vi "Binary Multiplication.vi"(10 "NUM 2 (Binary)":i32 format="%b", 11 "NUM 1 (Binary)":i32 format="%b") -> (3 "PRODUCT  (Binary)":i32 format="%b")   [LabVIEW 2020]
doc: "This VI will find a product between two Binary Numbers."
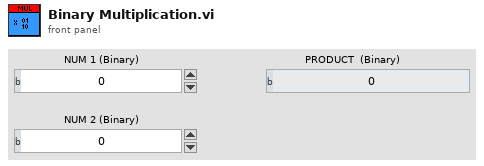
[diagram p1: front panel]
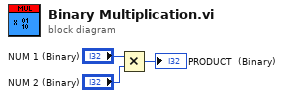
[diagram p0: block diagram]
diagram:
  n1 = Multiply(x="NUM 1 (Binary)", y="NUM 2 (Binary)") -> (x*y=→"PRODUCT  (Binary)":i32)
